vi "SineWaveSweep_Flows.vi"() -> ()   [LabVIEW 2016]
uses:
  <userlib>/Fluigent/Fluigent MFCS/FluigentMFCS_Full.llb/MFCS_EZ Detect.vi
  <userlib>/Fluigent/Fluigent MFCS/FluigentMFCS_Full.llb/MFCS_EZ Initialization.vi
  <userlib>/Fluigent/Fluigent MFCS/FluigentMFCS_Full.llb/MFCS_EZ Set Channel EV.vi
  <userlib>/Fluigent/Fluigent MFCS/FluigentMFCS_Full.llb/MFCS_EZ Close.vi
  <vilib>/measure/NI_MABase.lvlib
panel:
  out "Channel2Control":i16
  out "Waveform":dbl[](array[numeric])
  out "dt":u32=49
  in  "Vary Water?":bool
  in  "DeltaT":dbl=0.01
  in  "Period":dbl=10.0 format="%0.2p"
  in  "amplitude":dbl=10.0 format="%0.2p"
  in  "stop":bool
  in  "Valves":enum16{"1", "2", "3", "4", "5", "6", "7", "8"}[](array[ring])=[enum."6", enum."7"]
  in  "Pressure Channels":i16[](array[numeric])=[2, 3]
  in  "Manual Pressure Set":dbl[](array[numeric])=[630.0, 600.0]
  in  "Add Ctrl?":bool=TRUE
  in  "Boards":enum16{"A", "B", "C"}[](array[ring])=[enum."A", enum."A"]
  in  "Valves":enum16{"1", "2", "3", "4", "5", "6", "7", "8"}[](array[ring])=[enum."5", enum."4"]
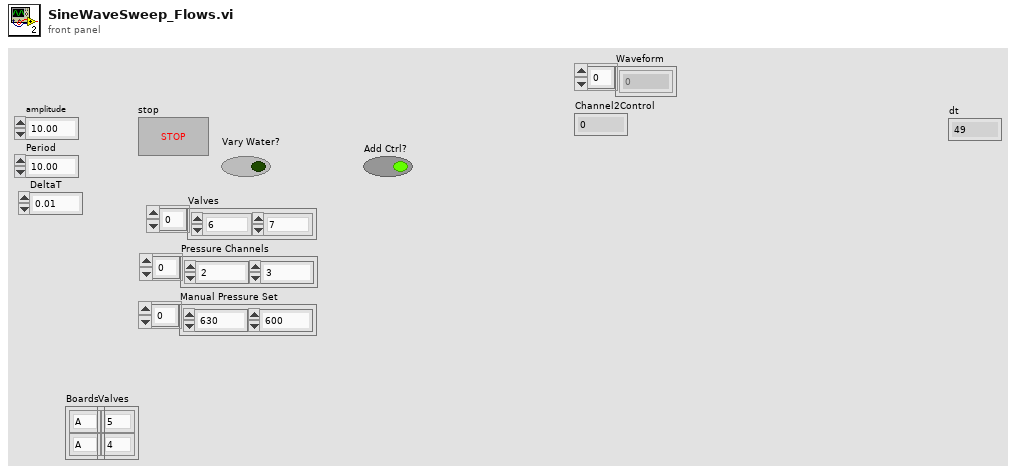
[diagram p1: front panel]
types:
  T1 = typedef "_EZmfcsSN.ctl" = u16
  T2 = typedef "_EZmfcsRefNum.ctl" = refnum<k1>
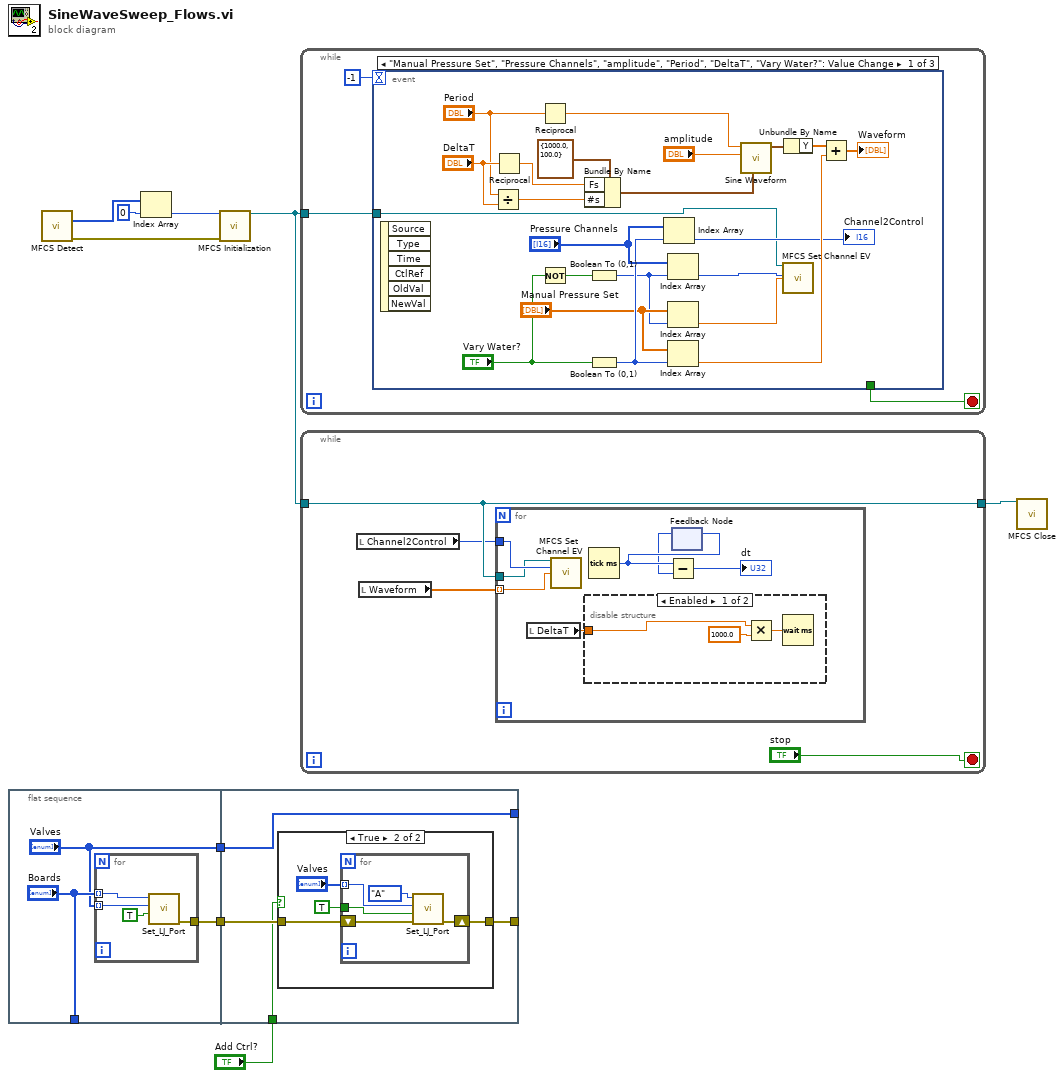
[diagram p0: block diagram]
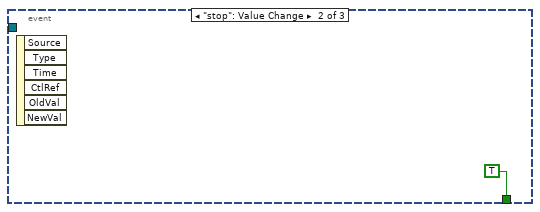
[diagram p2: hidden frame]
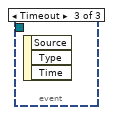
[diagram p3: hidden frame]
diagram:
  n1 = flat-sequence {
    tunnel: ["Boards"] -> _
    tunnel: [w12] -> w9
    tunnel: ["Valves"] -> w8
    tunnel: [w20] -> _
    tunnel: [w18] -> _
    tunnel: w9 -> [w19]
    tunnel: w8 -> [w20]
    tunnel: "Add Ctrl?" -> [w17]
    frame #0 {
      n2 = for {
        tunnel: "Valves" -> [w16] mode=indexing
        tunnel: "Boards" -> [w15] mode=indexing
        tunnel: [w13] -> w12
        n3 = call "Set_LJ_Port.vi"("State"=TRUE, "Channel"=w16, "Flowboard"=w15) -> ("error out"=w13:errorcluster)  [unwired: 8 in]
      }
    }
    frame #1 {
      n4 = case shown="True" w17 {
        tunnel: w19 -> [w21 w25]
        tunnel: [w21 w24] -> w18
        frame False {
        }
        frame True {
          n5 = for {
            tunnel: TRUE ("State") -> [w28]
            shift-right: [w29] -> w24
            shift-left: w25 -> [w30]
            tunnel: "Valves" -> [w27] mode=indexing
            n6 = call "Set_LJ_Port.vi"("error in"=w30, "State"=w28, "Channel"=w27, "Flowboard"=enum16{"A", "B", "C"}."A") -> ("error out"=w29:errorcluster)  [unwired: 7 in]
          }
        }
      }
    }
  }
  n7 = call-poly <userlib>:"MFCS Detect.vi"() -> ("[SN MFCS_EZ]"=w6:T1[], "error out"=w4:errorcluster)  [unwired: 14 in]
  n8 = Index Array(array=w6, index=0) -> (element=w5:T1)
  n9 = call-poly <userlib>:"MFCS Initialization.vi"("SN MFCS_EZ"=w5, "error in (no error)"=w4) -> ("MFCS_EZ"=w1:T2)  [unwired: 11 in, 2 out]
  n10 = while {
    tunnel: w1 -> [w33]
    stop <- w31 stop-if-true
    n11 = event shown="[0] \"Manual Pressure Set\", \"Pressure Channels\", \"amplitude\", \"Period\", \"DeltaT\", \"Vary Water?\": Value Change" {
      selector: _ -> [_ _ _]
      dyn-events: _ -> [_ _ _]
      timeout: -1 -> [_ _ _]
      tunnel: w33 -> [w37 _ _]
      tunnel: [_ TRUE _] -> w31
      event "Manual Pressure Set", "Pressure Channels", "amplitude", "Period", "DeltaT", "Vary Water?": Value Change {
        n12 = event-data() -> ()  [unwired: 1 in, 6 out]
        n13 = Divide(x="Period", y="DeltaT") -> (x/y=w45:dbl)
        n14 = Reciprocal(x="DeltaT") -> (1/x=w44:dbl)
        n15 = Reciprocal(x="Period") -> (1/x=w53:dbl)
        n16 = Not(x="Vary Water?") -> (.not. x?=w49:bool)
        n17 = Bundle By Name(cluster=cluster{"Fs":dbl, "#s":dbl} {"Fs"=1000.0, "#s"=100.0} ("sampling info"), "Fs"=w44, "#s"=w45) -> (w42:cluster{"Fs":dbl, "#s":dbl})
        n18 = Boolean To (0,1)(Boolean=w49) -> (0, 1=w35:i16)
        n19 = Boolean To (0,1)(Boolean="Vary Water?") -> (0, 1=w51:i16)
        n20 = Index Array(array="Pressure Channels", index=w51) -> (element=→"Channel2Control":i16)
        n21 = Index Array(array="Pressure Channels", index=w35) -> (element=w34:i16)
        n22 = Index Array(array="Manual Pressure Set", index=w35) -> (element=w36:dbl)
        n23 = Index Array(array="Manual Pressure Set", index=w51) -> (element=w46:dbl)
        n24 = call <vilib>:"Sine Waveform.vi"("sampling info"=w42, "amplitude"="amplitude", "frequency"=w53) -> ("signal out"=w43:waveform(dbl))  [unwired: 7 in, 1 out]
        n25 = call-poly <userlib>:"MFCS Set Channel EV.vi"("MFCS_EZ"=w37, "Channel Number (0=All)"=w34, "% EV"=w36) -> ()  [unwired: 11 in, 2 out]
        n26 = Unbundle By Name(w43) -> ("Y"=w47:dbl[])
        n27 = Add(x=w47, y=w46) -> (x+y=→"Waveform":dbl[])
      }
      event "stop": Value Change {
        n28 = event-data() -> ()  [unwired: 1 in, 6 out]
      }
      event Timeout {
        n29 = event-data() -> ()  [unwired: 1 in, 3 out]
      }
    }
  }
  n30 = while {
    tunnel: [w60] -> w2
    tunnel: w1 -> [w60]
    stop <- "stop" stop-if-true
    n31 = local read "Channel2Control"() -> (w57:i16)
    n32 = local read "Waveform"() -> (w58:dbl[])
    n33 = for {
      tunnel: w60 -> [w61]
      tunnel: w58 -> [w62] mode=indexing
      tunnel: w57 -> [w63]
      n34 = local read "DeltaT"() -> (w64:dbl)
      n35 = call-poly <userlib>:"MFCS Set Channel EV.vi"("MFCS_EZ"=w61, "Channel Number (0=All)"=w63, "% EV"=w62) -> ()  [unwired: 11 in, 2 out]
      n36 = disable-structure shown="Enabled" {
        disable-tunnel: w64 -> [w68 _]
        frame Enabled {
          n37 = Multiply(x=w68, y=1000.0) -> (x*y=w69:dbl)
          n38 = Wait (ms)(milliseconds to wait=w69) -> ()  [unwired: 1 out]
        }
        frame Disabled {
        }
      }
      n39 = Tick Count (ms)() -> (millisecond timer value=w66:u32)
      n40 = feedback #1() -> (w65:u32)  [unwired: 1 in]
      n41 = Subtract(x=w66, y=w65) -> (x-y=→"dt":u32)
      n42 = feedback-in #1(w66) -> ()
    }
  }
  n43 = call-poly <userlib>:"MFCS Close.vi"("MFCS_EZ"=w2) -> ()  [unwired: 14 in, 1 out]
